vi "JudgeOverForce.vi"(7 "MaxForceSpect":dbl, 8 "MaxForceUp":T1, 11 "MaxForceDown":T1) -> (0 "MaxForceOut 2":bool, 3 "MaxForceOut":bool, 4 "MaxForce":dbl)   [LabVIEW 2017]
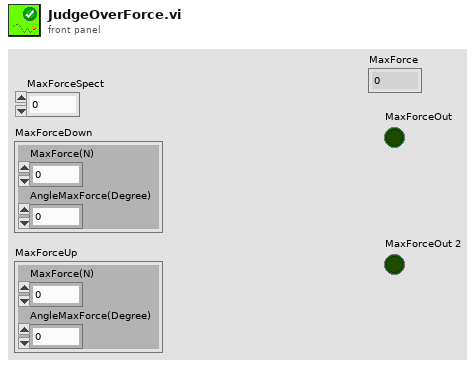
[diagram p1: front panel]
types:
  T1 = cluster{"MaxForce(N)":dbl, "AngleMaxForce(Degree)":dbl}
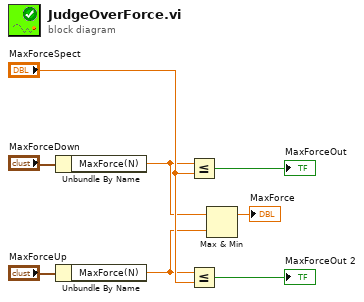
[diagram p0: block diagram]
diagram:
  n1 = Unbundle By Name("MaxForceDown") -> ("MaxForce(N)"=w3:dbl)
  n2 = Unbundle By Name("MaxForceUp") -> ("MaxForce(N)"=w2:dbl)
  n3 = Less Or Equal?(x=w3, y="MaxForceSpect") -> (x <= y?=→"MaxForceOut":bool)
  n4 = Less Or Equal?(x=w2, y="MaxForceSpect") -> (x <= y?=→"MaxForceOut 2":bool)
  n5 = Max & Min(x=w3, y=w2) -> (max(x,y)=→"MaxForce":dbl)  [unwired: 1 out]
